vi "Increment Last Nested Level Item.vi"(10 "offset":i32, 11 "nested level array":i32[](array[numeric])) -> (1 "previous nested level":i32, 2 "actual nested level":i32, 3 "deeper nested level":i32)   [LabVIEW 2014]
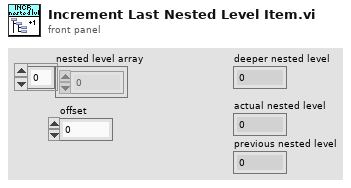
[diagram p1: front panel]
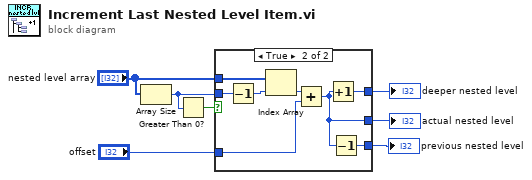
[diagram p0: block diagram]
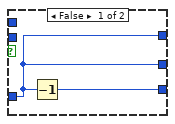
[diagram p2: hidden frame]
diagram:
  n1 = Array Size(array="nested level array") -> (size(s)=w5:i32)
  n2 = Greater Than 0?(x=w5) -> (x > 0?=w4:bool)
  n3 = case shown="True" w4 {
    tunnel: [w9 w17] -> w7
    tunnel: "nested level array" -> [_ w15]
    tunnel: w5 -> [_ w14]
    tunnel: [w9 w11] -> w3
    tunnel: [w8 w13] -> w2
    tunnel: "offset" -> [w9 w10]
    frame False {
      n4 = Decrement(x=w9) -> (x-1=w8:i32)
    }
    frame True {
      n5 = Decrement(x=w14) -> (x-1=w16:i32)
      n6 = Index Array(array=w15, index=w16) -> (element=w12:i32)
      n7 = Add(x=w12, y=w10) -> (x+y=w11:i32)
      n8 = Increment(x=w11) -> (x+1=w17:i32)
      n9 = Decrement(x=w11) -> (x-1=w13:i32)
    }
  }
  "deeper nested level" <- w7
  "actual nested level" <- w3
  "previous nested level" <- w2
